vi "process_storage_imaq.vi"() -> ()   [LabVIEW 2011, in "Fiberscope_library.lvlib"]
uses:
  Fiberscope_library.lvlib
  typedefs/control_process_state_cluster.ctl
  typedefs/control_process_state_enum.ctl
  typedefs/feedback_to_watchdog.ctl
  typedefs/feedback_from_process_enum.ctl
  typedefs/element_imaq_images_cluster.ctl
  <vilib>/vision/Image Controls.llb/IMAQ Image.ctl
  typedefs/all_scan_parameters_cluster.ctl
  typedefs/fiber_parameters_cluster.ctl
  fpga/typedefs/ramp_type_enum.ctl
  typedefs/spiral_parameters_cluster.ctl
  typedefs/run_parameters_cluster.ctl
  typedefs/run_mode_enum.ctl
  typedefs/acquisition_parameters_cluster.ctl
  typedefs/image_size_I32.ctl
  typedefs/smooth_coeffs_cluster.ctl
  typedefs/storage_parameters_cluster.ctl
  typedefs/mapping_corrections_cluster.ctl
  typedefs/pockels_corrections_cluster.ctl
panel:
  out "Local exit":bool
  out "Last saved image":string
  out "error out":errorcluster
  in  "error in":errorcluster
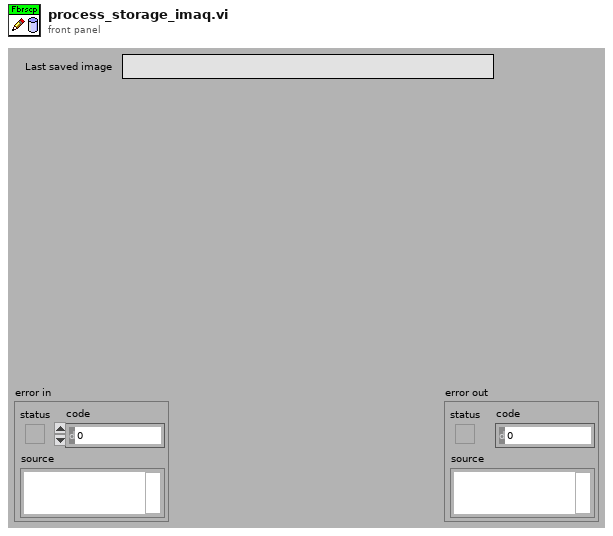
[diagram p1: front panel]
types:
  T1 = typedef "IMAQ Image.ctl" = refnum<image>
  T2 = typedef "Fiberscope_library.lvlib/element_imaq_images_cluster.ctl" = cluster{"Images":T1[], "#channels":i32, "Last element?":bool}
  T3 = typedef "Fiberscope_library.lvlib/feedback_to_watchdog.ctl" = cluster{"Feedback_from_process_enum":T4, "Process_name":string}
  T4 = typedef "Fiberscope_library.lvlib/feedback_from_process_enum.ctl" = enum16{"Has_initialised", "Changed_parameters", "Has_started", "Has_stopped", "Has_quitted", "Is_running", "Has_finished", "Custom"}
  T5 = typedef "Fiberscope_library.lvlib/control_process_state_cluster.ctl" = cluster{"Control_process_state_enum":T6, "variant":variant}
  T6 = typedef "Fiberscope_library.lvlib/control_process_state_enum.ctl" = enum16{"Init", "Quit", "Start", "Stop", "Change_parameters", "Running", "Finish", "Custom"}
  T7 = typedef "Fiberscope_library.lvlib/all_scan_parameters_cluster.ctl" = cluster{"Fiber parameters":T8, "Spiral parameters":T10, "Run parameters":T11, "Acquisition parameters":T13, "Fiber parameters pixel_mapper":T8, "Smooth_coeffs_cluster":T15, "Storage parameters":T16, "Mapping corrections":T17, "Pockels corrections":T18}
  T8 = typedef "Fiberscope_library.lvlib/fiber_parameters_cluster.ctl" = cluster{"Frequency":dbl, "Amplitude X":dbl, "Amplitude Y":dbl, "Initial Amplitude X":dbl, "Initial Amplitude Y":dbl, "Phase":dbl, "Ramp type":T9}
  T9 = typedef "ramp_type_enum.ctl" = enum8{"Linear", "Sine"}
  T10 = typedef "Fiberscope_library.lvlib/spiral_parameters_cluster.ctl" = cluster{"Imaging periods":dbl, "Settling periods":dbl, "Resting periods":dbl}
  T11 = typedef "Fiberscope_library.lvlib/run_parameters_cluster.ctl" = cluster{"Run mode":T12, "Averages per frame":u8, "No. of frames":u32}
  T12 = typedef "Fiberscope_library.lvlib/run_mode_enum.ctl" = enum16{"Continuous", "Single frame", "No. of frames"}
  T13 = typedef "Fiberscope_library.lvlib/acquisition_parameters_cluster.ctl" = cluster{"Cycles per pixel":u32, "Image size":T14, "Bidirectional acquisition":bool}
  T14 = typedef "Fiberscope_library.lvlib/image_size_I32.ctl" = i32
  T15 = typedef "Fiberscope_library.lvlib/smooth_coeffs_cluster.ctl" = cluster{"Coeff 1":dbl, "Coeff 2":dbl}
  T16 = typedef "Fiberscope_library.lvlib/storage_parameters_cluster.ctl" = cluster{"Autosave":bool, "Path":path}
  T17 = typedef "Fiberscope_library.lvlib/mapping_corrections_cluster.ctl" = cluster{"Phase increase":dbl, "Amplitude correction":dbl}
  T18 = typedef "Fiberscope_library.lvlib/pockels_corrections_cluster.ctl" = cluster{"Delay pixels":i32}
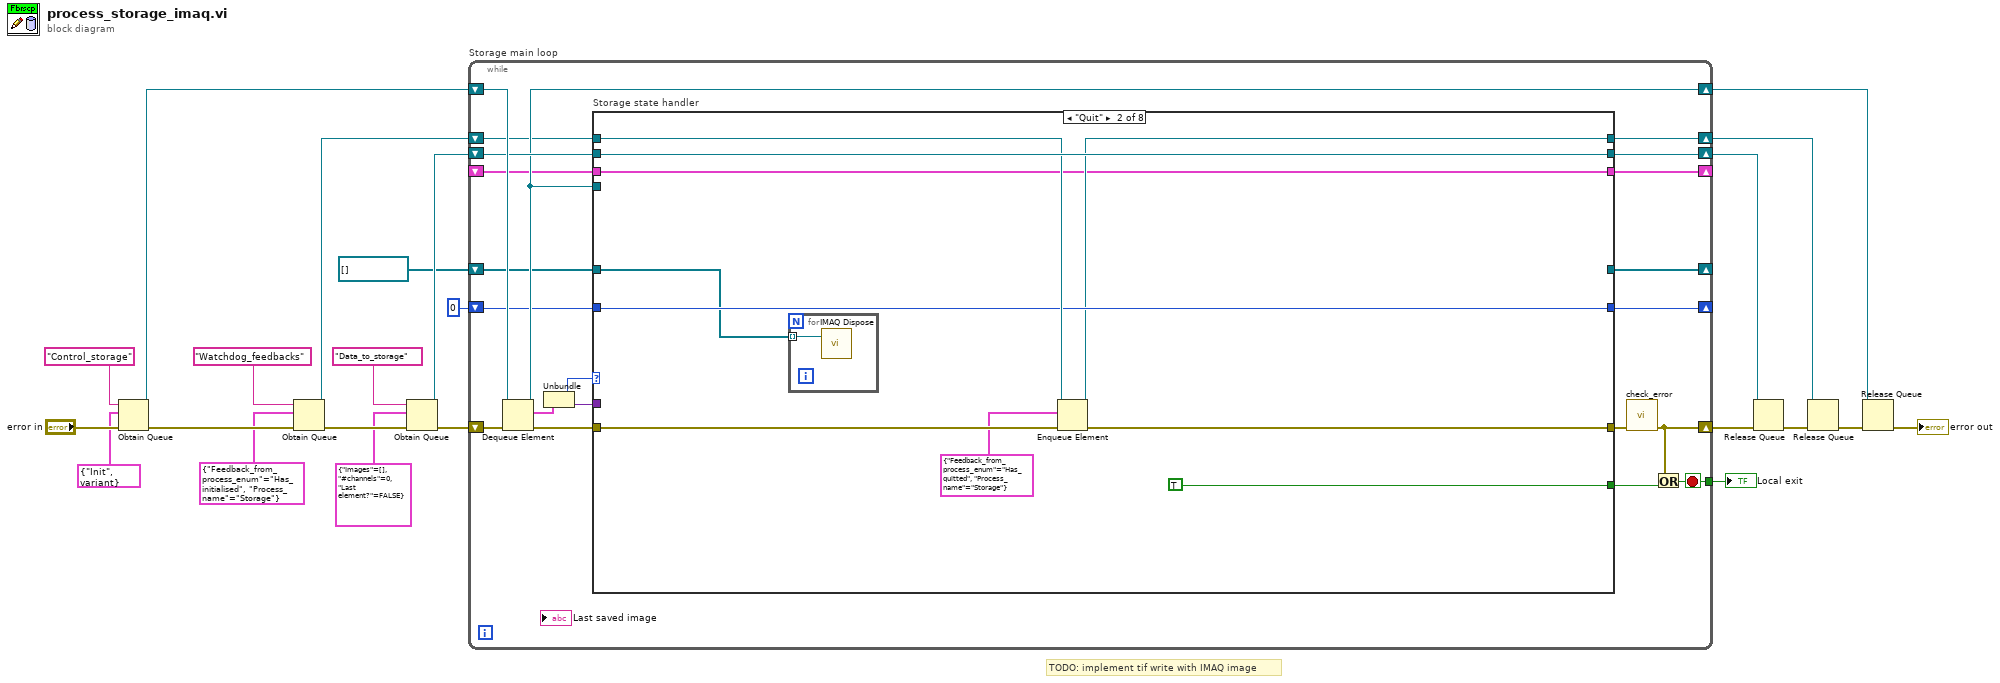
[diagram p0: block diagram]
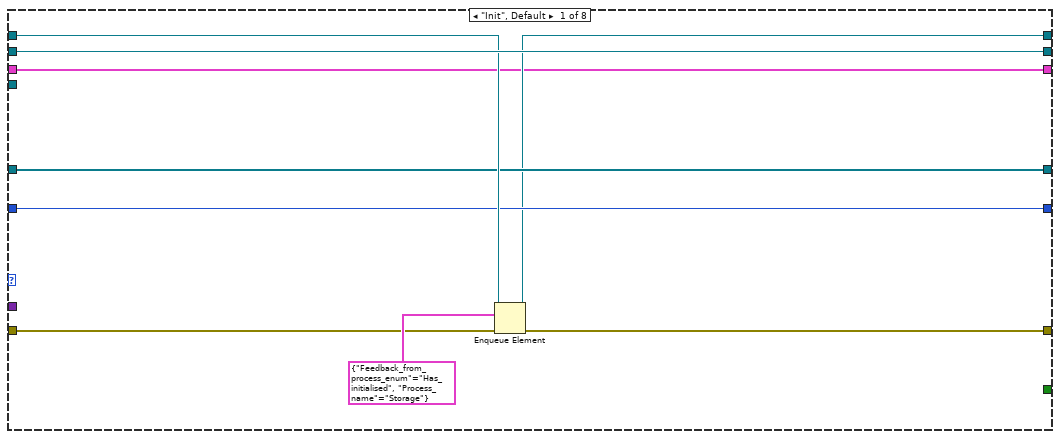
[diagram p2: hidden frame]
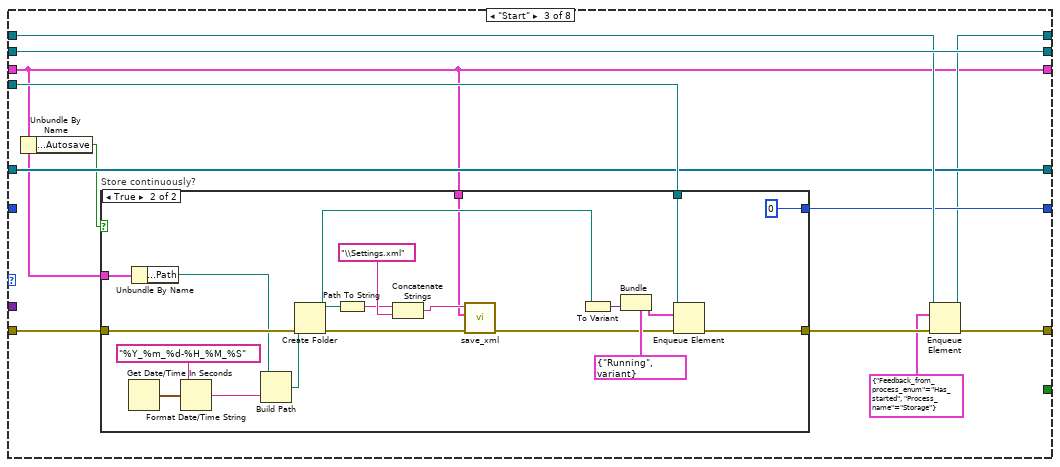
[diagram p3: hidden frame]
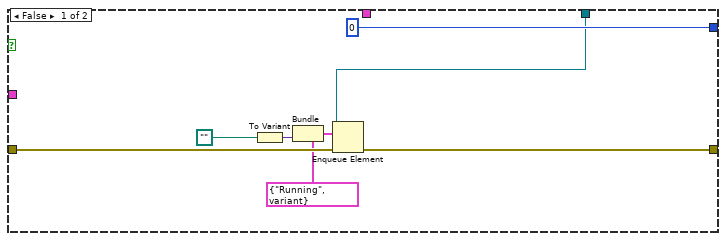
[diagram p4: hidden frame]
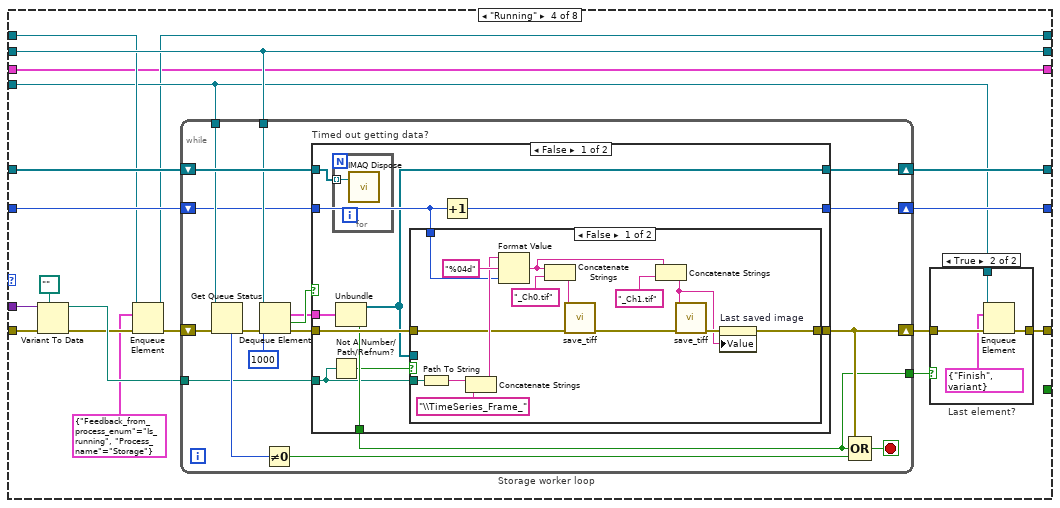
[diagram p5: hidden frame]
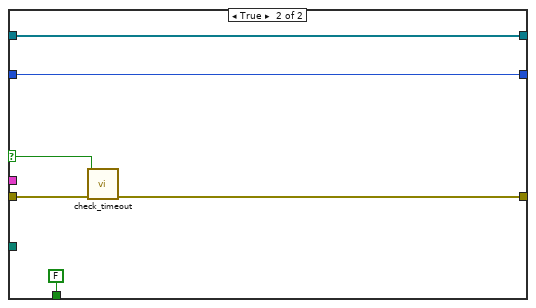
[diagram p8: hidden frame]
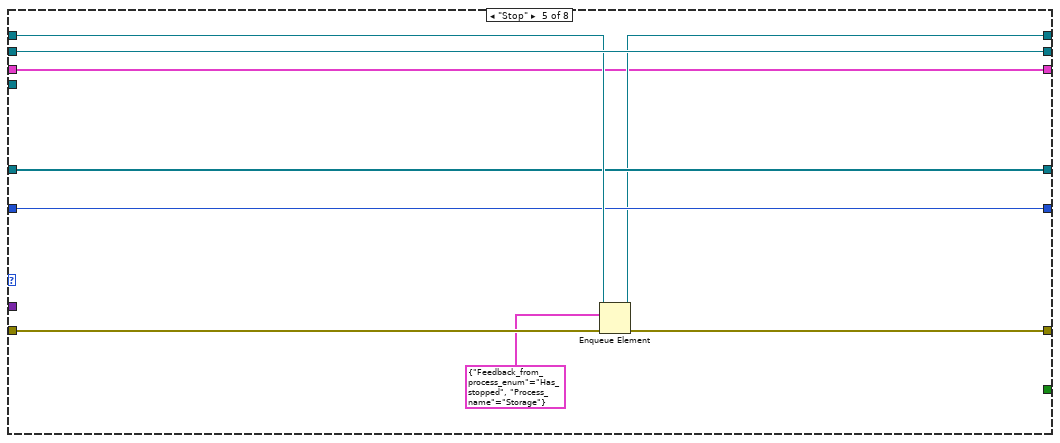
[diagram p9: hidden frame]
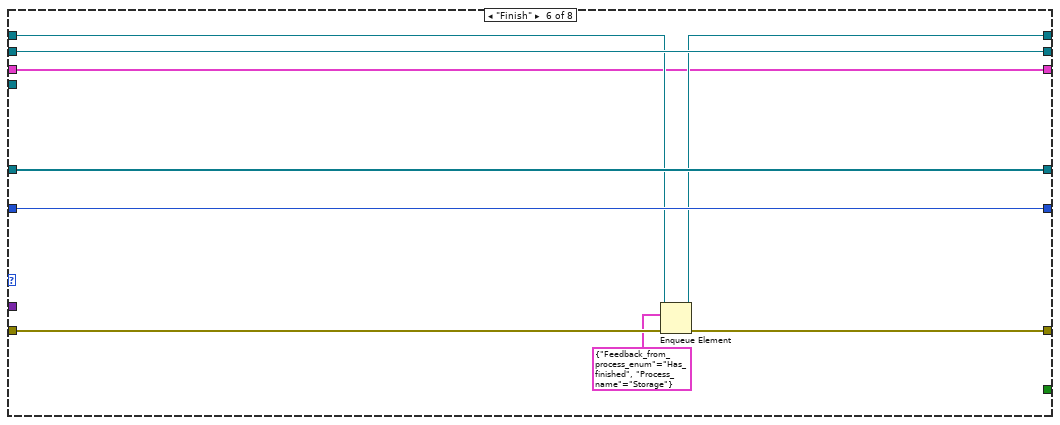
[diagram p10: hidden frame]
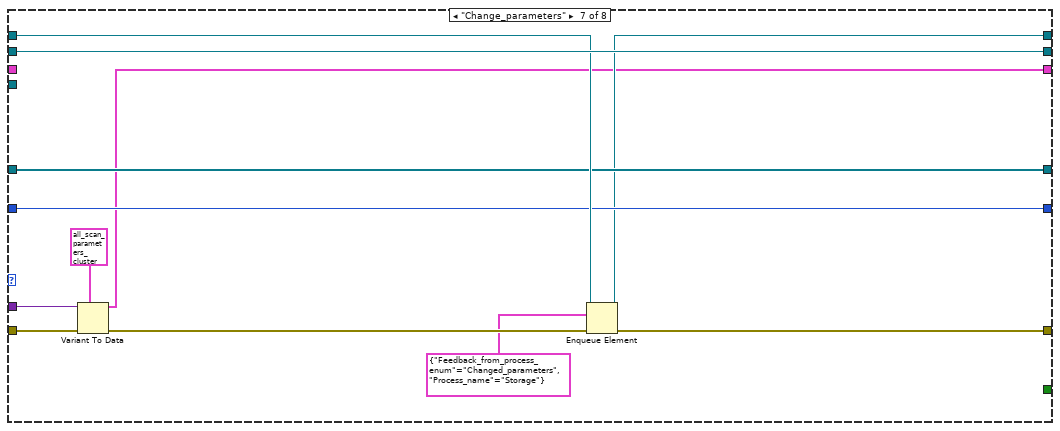
[diagram p11: hidden frame]
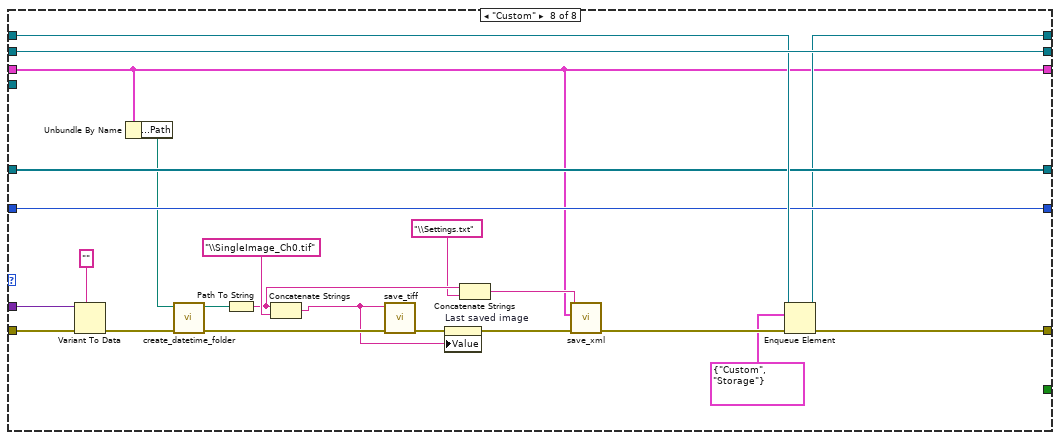
[diagram p12: hidden frame]
diagram:
  # "TODO: implement tif write with IMAQ image"
  n1 = Obtain Queue(name (unnamed)="Control_storage", element data type=T5 {"Control_process_state_enum"=enum."Init", "variant"=variant} ("Control_process_state_cluster"), error in (no error)="error in") -> (queue out=w8:refnum<queue>, error out=w7:errorcluster)  [unwired: 2 in, 1 out]
  n2 = Obtain Queue(name (unnamed)="Watchdog_feedbacks", element data type=T3 {"Feedback_from_process_enum"=enum."Has_initialised", "Process_name"="Storage"}, error in (no error)=w7) -> (queue out=w13:refnum<queue>, error out=w15:errorcluster)  [unwired: 2 in, 1 out]
  n3 = Obtain Queue(name (unnamed)="Data_to_storage", element data type=T2 {"Images"=[], "#channels"=0, "Last element?"=FALSE} ("Element_imaq_images_cluster"), error in (no error)=w15) -> (queue out=w19:refnum<queue>, error out=w20:errorcluster)  [unwired: 2 in, 1 out]
  n4 = while "Storage main loop" {
    shift-right: [w27] -> w18
    shift-left: w20 -> [w44]
    shift-right: [w35] -> w16
    shift-left: w8 -> [w43]
    shift-right: [w37] -> w17
    shift-left: w19 -> [w38]
    shift-right: [w26] -> w10
    shift-left: w13 -> [w33]
    shift-right: [w32] -> _
    shift-left: T1[] [] ("Images") -> [w31]
    tunnel: [w30] -> w9
    shift-right: [w29] -> _
    shift-left: 0 -> [w28]
    shift-right: [w25] -> _
    shift-left: _ -> [w24]
    stop <- w30 stop-if-true
    n5 = Dequeue Element(queue=w43, error in (no error)=w44) -> (queue out=w35:refnum<queue>, element=w41:T5, error out=w42:errorcluster)  [unwired: 1 in, 1 out]
    n6 = Unbundle(w41) -> ("Control_process_state_enum"=w40:T6, "variant"=w34:variant)
    n7 = case "Storage state handler" shown="\"Quit\"" w40 {
      tunnel: w42 -> [w45 w61 w73 w121 w187 w194 w208 w222]
      tunnel: [w52 w60 w69 w110 w186 w193 w205 w231] -> w36
      tunnel: [_ TRUE _ _ _ _ _ _] -> w39
      tunnel: w38 -> [w53 w62 w76 w116 w188 w197 w209 w232]
      tunnel: [w53 w62 w76 w116 w188 w197 w209 w232] -> w37
      tunnel: w35 -> [_ _ w74 w109 _ _ _ _]
      tunnel: w34 -> [_ _ _ w120 _ _ w207 w220]
      tunnel: w33 -> [w51 w59 w75 w112 w185 w192 w204 w230]
      tunnel: [w50 _ w72 w123 w184 w196 w203 w225] -> w32
      tunnel: w31 -> [w50 w54 w72 w122 w184 w196 w203 w225]
      tunnel: [w49 w58 w71 w117 w183 w195 w202 w226] -> w29
      tunnel: w28 -> [w49 w58 _ w118 w183 w195 w202 w226]
      tunnel: [w48 w57 w68 w107 w182 w191 w201 w214] -> w26
      tunnel: [w46 w55 w65 w105 w180 w189 w199 w210] -> w25
      tunnel: w24 -> [w46 w55 w65 w105 w180 w189 _ w210]
      frame "Init", Default {
        n8 = Enqueue Element(queue=w51, element=T3 {"Feedback_from_process_enum"=enum."Has_initialised", "Process_name"="Storage"}, error in (no error)=w45) -> (queue out=w48:refnum<queue>, error out=w52:errorcluster)  [unwired: 1 in, 1 out]
      }
      frame "Quit" {
        n9 = for {
          tunnel: w54 -> [w64] mode=indexing
          n10 = call "IMAQ Dispose"("Image"=w64) -> ()  [unwired: 5 in, 1 out]
        }
        n11 = Enqueue Element(queue=w59, element=T3 {"Feedback_from_process_enum"=enum."Has_quitted", "Process_name"="Storage"}, error in (no error)=w61) -> (queue out=w57:refnum<queue>, error out=w60:errorcluster)  [unwired: 1 in, 1 out]
      }
      frame "Start" {
        n12 = Unbundle By Name(w65) -> ("Storage parameters.Autosave"=w66:bool)
        n13 = case "Store continuously?" shown="True" w66 {
          tunnel: w74 -> [w81 w104]
          tunnel: w73 -> [w83 w99]
          tunnel: [0 0] -> w71
          tunnel: [w82 w97] -> w70
          tunnel: w65 -> [_ w85]
          tunnel: w65 -> [_ w87]
          frame False {
            n14 = To Variant(anything=path "") -> (Variant=w78:variant)
            n15 = Bundle(cluster=T5 {"Control_process_state_enum"=enum."Running", "variant"=variant} ("Control_process_state_cluster"), "variant"=w78) -> (w79:T5)  [unwired: 1 in]
            n16 = Enqueue Element(queue=w81, element=w79, error in (no error)=w83) -> (error out=w82:errorcluster)  [unwired: 1 in, 2 out]
          }
          frame True {
            n17 = Get Date/Time In Seconds() -> (seconds since 1Jan1904=w103:timestamp)
            n18 = Unbundle By Name(w87) -> ("Storage parameters.Path"=w86:path)
            n19 = Format Date/Time String(time format string (%c)="%Y_%m_%d-%H_%M_%S", seconds (now)=w103) -> (date/time string=w102:string)  [unwired: 1 in]
            n20 = Build Path(base path=w86, name or relative path=w102) -> (appended path=w100:path)
            n21 = Create Folder(path (use dialog)=w100, error in=w99) -> (created path=w92:path, error out=w89:errorcluster)  [unwired: 1 in, 1 out]
            n22 = Path To String(path=w92) -> (string=w91:string)
            n23 = Concatenate Strings(w91, "\\Settings.xml" ("string")) -> (w90:string)
            n24 = call "save_xml.vi"("error in"=w89, "All scan parameters"=w85, "Path"=w90) -> ("error out"=w88:errorcluster)  [unwired: 8 in]
            n25 = To Variant(anything=w92) -> (Variant=w96:variant)
            n26 = Bundle(cluster=T5 {"Control_process_state_enum"=enum."Running", "variant"=variant} ("Control_process_state_cluster"), "variant"=w96) -> (w95:T5)  [unwired: 1 in]
            n27 = Enqueue Element(queue=w104, element=w95, error in (no error)=w88) -> (error out=w97:errorcluster)  [unwired: 1 in, 2 out]
          }
        }
        n28 = Enqueue Element(queue=w75, element=T3 {"Feedback_from_process_enum"=enum."Has_started", "Process_name"="Storage"}, error in (no error)=w70) -> (queue out=w68:refnum<queue>, error out=w69:errorcluster)  [unwired: 1 in, 1 out]
      }
      frame "Running" {
        n29 = Variant To Data(error in=w121, type=path "" ("Path"), Variant=w120) -> (data=w115:path, error out=w114:errorcluster)
        n30 = Enqueue Element(queue=w112, element=T3 {"Feedback_from_process_enum"=enum."Is_running", "Process_name"="Storage"}, error in (no error)=w114) -> (queue out=w107:refnum<queue>, error out=w113:errorcluster)  [unwired: 1 in, 1 out]
        n31 = while "Storage worker loop" {
          shift-right: [w130] -> w111
          shift-left: w113 -> [w146]
          shift-right: [w137] -> w123
          shift-left: w122 -> [w136]
          shift-right: [w131] -> w117
          shift-left: w118 -> [w132]
          tunnel: w109 -> [w135]
          tunnel: w116 -> [w134]
          tunnel: w115 -> [w133]
          tunnel: [w129] -> w108
          stop <- w143 stop-if-true
          n32 = Get Queue Status(queue=w135, error in (no error)=w146) -> (error out=w145:errorcluster, # elements in queue=w144:i32)  [unwired: 1 in, 6 out]
          n33 = Dequeue Element(queue=w134, timeout in ms (-1)=1000, error in (no error)=w145) -> (element=w138:T2, timed out?=w139:bool, error out=w140:errorcluster)  [unwired: 1 out]
          n34 = Not Equal To 0?(x=w144) -> (x != 0?=w142:bool)
          n35 = case "Timed out getting data?" shown="False" w139 {
            selector: w139 -> [_ w177]
            tunnel: w140 -> [w154 w179]
            tunnel: [w153 w178] -> w130
            tunnel: w138 -> [w152 _]
            tunnel: [w148 w176] -> w137
            tunnel: w136 -> [w147 w176]
            tunnel: w133 -> [w150 _]
            tunnel: w132 -> [w156 w175]
            tunnel: [w155 w175] -> w131
            tunnel: [w151 FALSE ("Last element?")] -> w129
            frame False {
              n36 = Not A Number/Path/Refnum?(number/path/refnum=w150) -> (NaN/Path/Refnum?=w149:bool)
              n37 = for {
                tunnel: w147 -> [w157] mode=indexing
                n38 = call "IMAQ Dispose"("Image"=w157) -> ()  [unwired: 5 in, 1 out]
              }
              n39 = Unbundle(w152) -> ("Images"=w148:T1[], "Last element?"=w151:bool)  [unwired: 1 out]
              n40 = case shown="False" w149 {
                tunnel: w150 -> [w170 _]
                tunnel: w156 -> [w166 _]
                tunnel: w154 -> [w165 w173]
                tunnel: [w164 w173] -> w153
                tunnel: w148 -> [_ _]
                frame False {
                  n41 = Path To String(path=w170) -> (string=w172:string)
                  n42 = Concatenate Strings(w172, "\\TimeSeries_Frame_" ("string")) -> (w168:string)
                  n43 = Format Value(string ("")=w168, format string="%04d", value (0)=w166) -> (output string=w160:string)
                  n44 = Concatenate Strings(w160, "_Ch0.tif" ("string")) -> (w163:string)
                  n45 = call "save_tiff.vi"("error in (no error)"=w165, "Path"=w163) -> ("error out"=w162:errorcluster)  [unwired: 9 in]
                  n46 = Concatenate Strings(w160, "_Ch1.tif" ("string")) -> (w158:string)
                  n47 = call "save_tiff.vi"("error in (no error)"=w162, "Path"=w158) -> ("error out"=w161:errorcluster)  [unwired: 9 in]
                  n48 = property on="Last saved image" class="Str"(error in=w161, "Value"=w158) -> (error out=w164:errorcluster)  [unwired: 1 in, 1 out]
                }
                frame True {
                  # "No valid path provided\n-> do not store continuously!"
                }
              }
              n49 = Increment(x=w156) -> (x+1=w155:i32)
            }
            frame True {
              n50 = call "check_timeout.vi"("error in"=w179, "Timeout?"=w177) -> ("error out"=w178:errorcluster)  [unwired: 9 in]
            }
          }
          n51 = Compound Arithmetic op=OR(w130, w129, w142) -> (w143:bool)
        }
        n52 = case "Last element?" shown="True" w108 {
          tunnel: w111 -> [w124 w128]
          tunnel: [w124 w127] -> w110
          tunnel: w109 -> [_ w126]
          frame False {
          }
          frame True {
            n53 = Enqueue Element(queue=w126, element=T5 {"Control_process_state_enum"=enum."Finish", "variant"=variant} ("Control_process_state_cluster"), error in (no error)=w128) -> (error out=w127:errorcluster)  [unwired: 1 in, 2 out]
          }
        }
      }
      frame "Stop" {
        n54 = Enqueue Element(queue=w185, element=T3 {"Feedback_from_process_enum"=enum."Has_stopped", "Process_name"="Storage"}, error in (no error)=w187) -> (queue out=w182:refnum<queue>, error out=w186:errorcluster)  [unwired: 1 in, 1 out]
      }
      frame "Finish" {
        n55 = Enqueue Element(queue=w192, element=T3 {"Feedback_from_process_enum"=enum."Has_finished", "Process_name"="Storage"}, error in (no error)=w194) -> (queue out=w191:refnum<queue>, error out=w193:errorcluster)  [unwired: 1 in, 1 out]
      }
      frame "Change_parameters" {
        n56 = Variant To Data(error in=w208, type=T7 {"Fiber parameters"={"Frequency"=100.0, "Amplitude X"=0.0, "Amplitude Y"=0.0, "Initial Amplitude X"=0.0, "Initial Amplitude Y"=0.0, "Phase"=0.0, "Ramp type"=enum."Linear"}, "Spiral parameters"={"Imaging periods"=1.0, "Settling periods"=1.0, "Resting periods"=1.0}, "Run parameters"={"Run mode"=enum."Continuous", "Averages per frame"=1, "No. of frames"=1}, "Acquisition parameters"={"Cycles per pixel"=1, "Image size"=128, "Bidirectional acquisition"=FALSE}, "Fiber parameters pixel_mapper"={"Frequency"=100.0, "Amplitude X"=0.0, "Amplitude Y"=0.0, "Initial Amplitude X"=0.0, "Initial Amplitude Y"=0.0, "Phase"=0.0, "Ramp type"=enum."Linear"}, "Smooth_coeffs_cluster"={"Coeff 1"=0.0, "Coeff 2"=0.0}, "Storage parameters"={"Autosave"=FALSE, "Path"=path "D:/"}, "Mapping corrections"={"Phase increase"=0.0, "Amplitude correction"=0.0}, "Pockels corrections"={"Delay pixels"=0}} ("All scan parameters"), Variant=w207) -> (data=w199:T7, error out=w206:errorcluster)
        n57 = Enqueue Element(queue=w204, element=T3 {"Feedback_from_process_enum"=enum."Changed_parameters", "Process_name"="Storage"}, error in (no error)=w206) -> (queue out=w201:refnum<queue>, error out=w205:errorcluster)  [unwired: 1 in, 1 out]
      }
      frame "Custom" {
        n58 = Variant To Data(error in=w222, type="" ("Comment"), Variant=w220) -> (error out=w221:errorcluster)  [unwired: 1 out]
        n59 = Unbundle By Name(w210) -> ("Storage parameters.Path"=w211:path)
        n60 = call "create_datetime_folder.vi"("error in (no error)"=w221, "Path"=w211) -> ("error out"=w228:errorcluster, "created path"=w229:path)  [unwired: 8 in]
        n61 = Path To String(path=w229) -> (string=w219:string)
        n62 = Concatenate Strings(w219, "\\SingleImage_Ch0.tif" ("string")) -> (w223:string)
        n63 = call "save_tiff.vi"("error in (no error)"=w228, "Path"=w223) -> ("error out"=w224:errorcluster)  [unwired: 9 in]
        n64 = property on="Last saved image" class="Str"(error in=w224, "Value"=w223) -> (error out=w217:errorcluster)  [unwired: 1 in, 1 out]
        n65 = Concatenate Strings(w219, "\\Settings.txt" ("string")) -> (w215:string)
        n66 = call "save_xml.vi"("error in"=w217, "All scan parameters"=w210, "Path"=w215) -> ("error out"=w216:errorcluster)  [unwired: 8 in]
        n67 = Enqueue Element(queue=w230, element=T3 {"Feedback_from_process_enum"=enum."Custom", "Process_name"="Storage"}, error in (no error)=w216) -> (queue out=w214:refnum<queue>, error out=w231:errorcluster)  [unwired: 1 in, 1 out]
      }
    }
    n68 = call "check_error.vi"("error in"=w36) -> ("error out"=w27:errorcluster)  [unwired: 10 in]
    n69 = Or(x=w27, y=w39) -> (x .or. y?=w30:bool)
  }
  "Local exit" <- w9
  n70 = Release Queue(queue=w17, error in (no error)=w18) -> (error out=w12:errorcluster)  [unwired: 1 in, 2 out]
  n71 = Release Queue(queue=w10, error in (no error)=w12) -> (error out=w11:errorcluster)  [unwired: 1 in, 2 out]
  n72 = Release Queue(queue=w16, error in (no error)=w11) -> (error out=→"error out":errorcluster)  [unwired: 1 in, 2 out]
